vi "Buzzer.vi"() -> ()   [LabVIEW 2022 SP3]
uses:
  <vilib>/DAQmx/write.llb/DAQmx Write (Digital Bool 1Line 1Point).vi
  <vilib>/DAQmx/miscellaneous.llb/DAQmx Fill In Error Info.vi
panel:
  in  "True":bool
  in  "False":bool
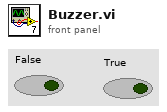
[diagram p1: front panel]
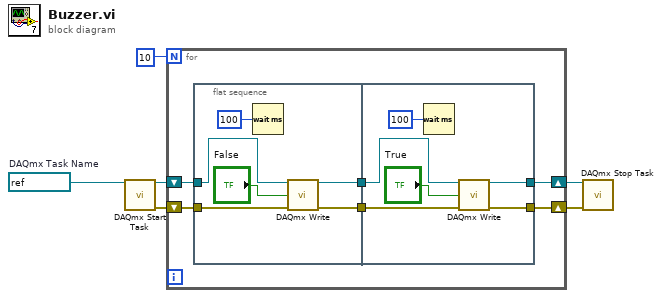
[diagram p0: block diagram]
diagram:
  w6 = refnum<k21> "Buzzer"  # DAQmx Task Name
  n1 = call <vilib>:"DAQmx Start Task.vi"("task/channels in"=w6) -> ("task out"=w4:refnum<k21>, "error out"=w5:errorcluster)  [unwired: 13 in]
  n2 = for {
    N: 10 -> [_]
    shift-right: [w7] -> w2
    shift-left: w5 -> [w10]
    shift-right: [w8] -> w3
    shift-left: w4 -> [w9]
    n3 = flat-sequence {
      tunnel: w10 -> [w18]
      tunnel: w9 -> [w17]
      tunnel: [w16] -> w12
      tunnel: [w15] -> w11
      tunnel: w12 -> [w23]
      tunnel: w11 -> [w22]
      tunnel: [w21] -> w8
      tunnel: [w20] -> w7
      frame #0 {
        n4 = Wait (ms)(milliseconds to wait=100) -> ()  [unwired: 1 out]
        n5 = call-poly <vilib>:"DAQmx Write.vi"("task/channels in"=w17, "data"="False", "error in"=w18) -> ("task out"=w16:refnum<k21>, "error out"=w15:errorcluster)  [unwired: 10 in, 1 out]
      }
      frame #1 {
        n6 = Wait (ms)(milliseconds to wait=100) -> ()  [unwired: 1 out]
        n7 = call-poly <vilib>:"DAQmx Write.vi"("task/channels in"=w23, "data"="True", "error in"=w22) -> ("task out"=w21:refnum<k21>, "error out"=w20:errorcluster)  [unwired: 10 in, 1 out]
      }
    }
  }
  n8 = call <vilib>:"DAQmx Stop Task.vi"("task/channels in"=w3, "error in"=w2) -> ()  [unwired: 12 in, 2 out]
